vi "Get Target Elevator Angle.vi"(10 "Robot Mode":T2, 11 "Shooter Mode":T1(ring)) -> (3 "Target Angle":dbl)   [LabVIEW 2013]
uses:
  <vilib>/Rock Robotics/WPI/DriverStation/WPI_DriverStationRobotMode2.ctl
  Robot Global Data.vi
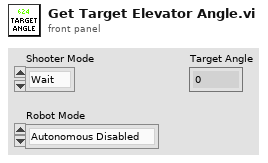
[diagram p1: front panel]
types:
  T1 = enum16{"Wait", "Adjust Angle", "Warmup Shooter", "Fire", "Feeding", "Neutral Angle"}
  T2 = typedef "WPI_DriverStationRobotMode2.ctl" = enum16{"Autonomous Disabled", "Autonomous Enabled", "Teleop Disabled", "Teleop Enabled", "Timeout", "Finish", "Test Disabled", "Test Enabled"}
  T3 = typedef "UDP Dashboard Packet.ctl" = cluster{"Feed Angle":dbl, "Neutral Angle":dbl, "Autonomous Setpoints":T4, "Auto Shift":T5, "Elevator Angle Offset":dbl, "Potentiometer Angle":cluster{"Pot M":dbl, "Pot B":dbl}, "Shoot Setpoints":cluster{"Vision":T6, "Back Corner":T6, "Front":T6, "Front Corner":T6, "Half Court":T6, "Full Court":T6, "Pyramid":T6}, "Halo Drive":T7, "Auto Speed Constants":T8, "Shooting Delays":cluster{"Unjam On":dbl, "Unjam Off":dbl, "Flipper On":dbl, "Flipper Off":dbl, "Hopper Up":dbl}, "Left Roller Pwr":dbl, "Right Roller Pwr":dbl, "Elevator PID Gains":cluster{"proportional gain (Kc)":dbl, "integral time (Ti, min)":dbl, "derivative time (Td, min)":dbl}, "Elevator PID Output Range":cluster{"output high":dbl, "output low":dbl}, "Elevator Angle Tolerance":dbl, "Toggle Ears Delay":dbl, "Toggle Ears Distance":dbl, "Unjam Servo Angle":dbl, "Auton Steer PID gains":cluster{"proportional gain (Kc)":dbl, "integral time (Ti, min)":dbl, "derivative time (Td, min)":dbl}, "Auton Steer output range":cluster{"output high":dbl, "output low":dbl}, "Auto Reverse Speed":dbl, "Auto Stop Throttle":dbl, "Auto Stop Duration":dbl, "Spin output range":cluster{"output high":dbl, "output low":dbl}, "Spin PID gains":cluster{"proportional gain (Kc)":dbl, "integral time (Ti, min)":dbl, "derivative time (Td, min)":dbl}, "Auto-Center Line":T9, "Auton Distance PID gains Low Gear":cluster{"proportional gain (Kc)":dbl, "integral time (Ti, min)":dbl, "derivative time (Td, min)":dbl}, "Auton Distance output range":cluster{"output high":dbl, "output low":dbl}, "Auton Distance Threshold":dbl, "Auton Velocity Cutoff":dbl, "Auton Distance output range Center Line":cluster{"output high":dbl, "output low":dbl}, "Auton Distance PID gains High Gear":cluster{"proportional gain (Kc)":dbl, "integral time (Ti, min)":dbl, "derivative time (Td, min)":dbl}}
  T4 = typedef "Autonomous Setpoints.ctl" = cluster{"Shoot Angle 1":dbl, "Initial Delay":dbl, "Disc Count 1":dbl, "Shoot Time 1":dbl, "Distance 1":dbl, "Two Disc Distance 1":dbl, "Distance 2":dbl, "Two Disc Distance 2":dbl, "Distance 3":dbl, "Two Disc Distance 3":dbl, "Shoot Angle 3":dbl, "Disc Count 3":dbl, "Shoot Time 3":dbl, "Distance 4":dbl, "Two Disc Distance 4":dbl, "Low Gear":bool, "Shoot 1 Post Delay":dbl}
  T5 = typedef "Auto Shift Settings.ctl" = cluster{"Enabled":bool, "Upshift Speed":dbl, "Downshift Speed":dbl, "Upshift Throttle":dbl, "Turn Power Diff":dbl, "Motor Limit":dbl, "Encoder Limit":dbl}
  T6 = typedef "Shoot Profile.ctl" = cluster{"Pre RPM":dbl, "Main RPM":dbl, "Angle":dbl}
  T7 = typedef "Halo Drive.ctl" = cluster{"Gains":cluster{"Quickturn_Sens_Low":dbl, "Quickturn_Sens_High":dbl, "Speedturn_Sens_Low":dbl, "Speedturn_Sens_High":dbl}, "QuickTurn Const":dbl, "Loading Throttle Limit":dbl}
  T8 = typedef "Auto Speed Constants.ctl" = cluster{"Slowing Distance":dbl, "High Speed":dbl, "Rampup Time":dbl, "Low Speed":dbl, "High Speed (Reverse)":dbl}
  T9 = typedef "Autonomous Center Line Setpoints.ctl" = cluster{"Arc Turn x-axis":dbl, "Arc Turn y-axis":dbl, "Arc Turn Distance":dbl, "Distance 1":dbl, "Two Disc Distance 1":dbl, "Distance 2":dbl, "Two Disc Distance 2":dbl, "Spin Angle":dbl, "Spin Angle tolerance":dbl, "Spin y-axis":dbl, "Spin Distance":dbl, "Center Line Enabled":bool, "Distance 3":dbl, "Two Disc Distance 3":dbl, "Spin Angle 2":dbl, "Spin Angle tolerance 2":dbl, "Spin y-axis 2":dbl, "Spin Distance 2":dbl, "Shoot Angle 1":dbl, "Disc Count 1":dbl, "Shoot Time 1":dbl, "Shoot Angle 3":dbl, "Disc Count 3":dbl, "Shoot Time 3":dbl, "Low Gear":bool}
  T10 = typedef "Autonomous Commands.ctl" = cluster{"Load":bool, "Warmup":bool, "Low Gear":bool, "Shoot Angle":dbl, "Azimuth":bool, "Elevator":bool, "Neutral Angle":dbl, "Two Discs":bool, "Shoot":bool}
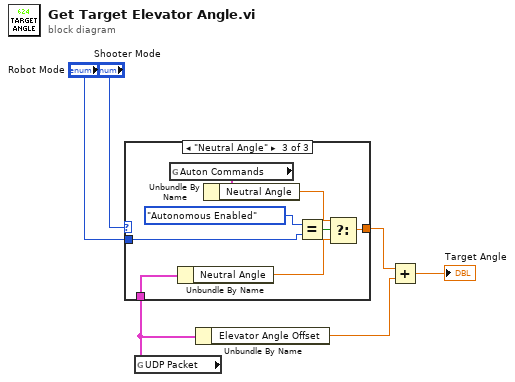
[diagram p0: block diagram]
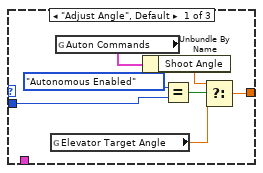
[diagram p2: hidden frame]
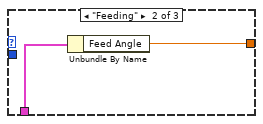
[diagram p3: hidden frame]
diagram:
  n1 = global read "Robot Global Data.vi" "UDP Packet"() -> (w6:T3)
  n2 = case shown="\"Neutral Angle\"" "Shooter Mode" {
    tunnel: [w8 w15 w21] -> w3
    tunnel: "Robot Mode" -> [w7 _ w19]
    tunnel: w6 -> [_ w14 w16]
    frame "Adjust Angle", Default {
      n3 = global read "Robot Global Data.vi" "Elevator Target Angle"() -> (w9:dbl)
      n4 = global read "Robot Global Data.vi" "Auton Commands"() -> (w11:T10)
      n5 = Unbundle By Name(w11) -> ("Shoot Angle"=w10:dbl)
      n6 = Equal?(x=WPI_DriverStationRobotMode2."Autonomous Enabled", y=w7) -> (x = y?=w12:bool)
      n7 = Select(t=w10, s=w12, f=w9) -> (s? t:f=w8:dbl)
    }
    frame "Feeding" {
      n8 = Unbundle By Name(w14) -> ("Feed Angle"=w15:dbl)
    }
    frame "Neutral Angle" {
      n9 = global read "Robot Global Data.vi" "Auton Commands"() -> (w22:T10)
      n10 = Unbundle By Name(w16) -> ("Neutral Angle"=w17:dbl)
      n11 = Unbundle By Name(w22) -> ("Neutral Angle"=w20:dbl)
      n12 = Equal?(x=WPI_DriverStationRobotMode2."Autonomous Enabled" ("y"), y=w19) -> (x = y?=w23:bool)
      n13 = Select(t=w20, s=w23, f=w17) -> (s? t:f=w21:dbl)
    }
  }
  n14 = Unbundle By Name(w6) -> ("Elevator Angle Offset"=w5:dbl)
  n15 = Add(x=w3, y=w5) -> (x+y=→"Target Angle":dbl)
